vi "AlazarFFTGetMaxTriggerRepeatRate.vi"(4 "error in (no error)":errorcluster, 6 "FFT Size":u32, 7 "DSP Handle":u64) -> (0 "error out":errorcluster, 1 "Return Code":u32, 2 "Trigger Repeat Rate":dbl, 3 "DSP Handle 2":u64)   [LabVIEW 2009]
doc: "Get the total number of board systems detected."
uses:
  ATSApi.dll
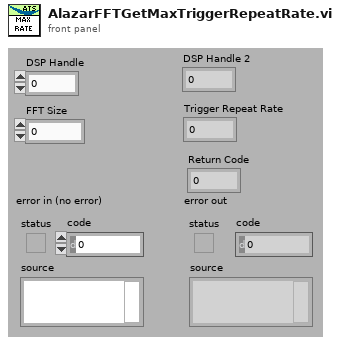
[diagram p1: front panel]
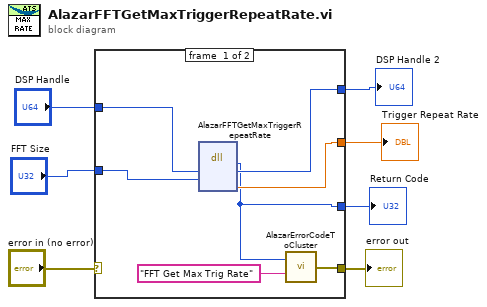
[diagram p0: block diagram]
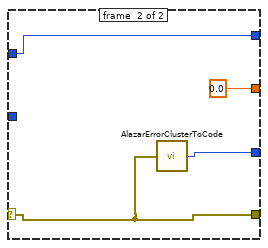
[diagram p2: hidden frame]
diagram:
  n1 = case shown="No Error" "error in (no error)" {
    selector: "error in (no error)" -> [_ w18]
    tunnel: [w10 w18] -> w6
    tunnel: "FFT Size" -> [w14 _]
    tunnel: "DSP Handle" -> [w13 w15]
    tunnel: [w12 w15] -> w3
    tunnel: [w8 w17] -> w2
    tunnel: [w9 0.0] -> w1
    frame #0 {
      n2 = dll-call lib="ATSApi.dll" fn="AlazarFFTGetMaxTriggerRepeatRate"("handle"=w13, "fft_size"=w14) -> ("return type"=w8:u32, "handle"=w12:u64, "rate"=w9:dbl)  [unwired: 5 in, 2 out]
      n3 = call "AlazarErrorCodeToCluster.vi"("Message"="FFT Get Max Trig Rate", "Error Code"=w8) -> ("error out"=w10:errorcluster)
    }
    frame #1 {
      n4 = call "AlazarErrorClusterToCode.vi"("error in (no error)"=w18) -> ("Error Code"=w17:u32)
    }
  }
  "error out" <- w6
  "Trigger Repeat Rate" <- w1
  "DSP Handle 2" <- w3
  "Return Code" <- w2
